vi "BESS reconnect.vi"() -> (1 "failure_flag 2":bool)   [LabVIEW 2016]
uses:
  Communication/Global communication.vi
  Communication/Global communication output.vi
panel:
  in  "ready?":bool
  in  "i>=20?":bool
  in  "=1?":bool
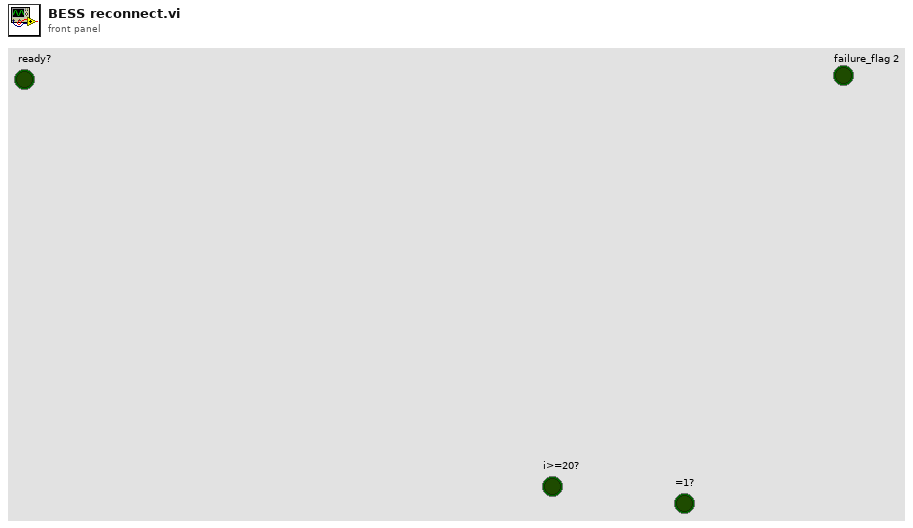
[diagram p1: front panel]
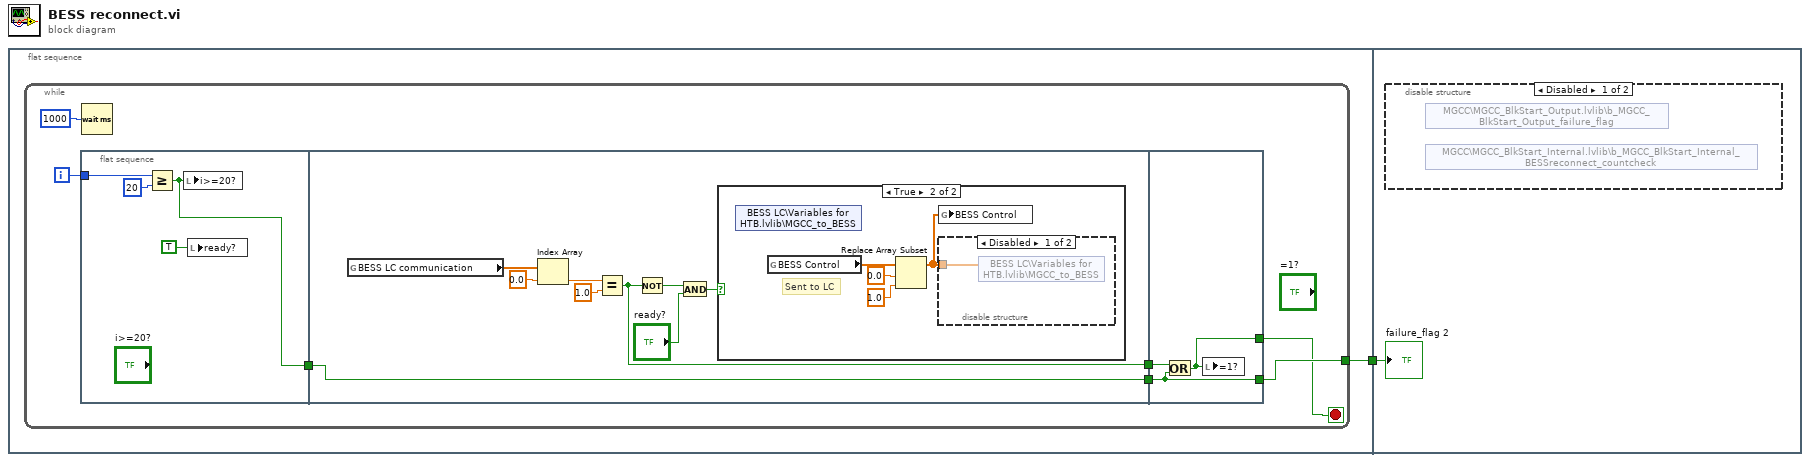
[diagram p0: block diagram]
diagram:
  n1 = flat-sequence {
    tunnel: [w2] -> w1
    tunnel: w1 -> [w31]
    frame #0 {
      n2 = while {
        tunnel: [w4] -> w2
        i -> [w8]
        stop <- w3 stop-if-true
        n3 = flat-sequence {
          tunnel: w8 -> [w13]
          tunnel: [w10] -> w7
          tunnel: w7 -> [w21]
          tunnel: [w21] -> w6
          tunnel: [w17] -> w5
          tunnel: w6 -> [w29]
          tunnel: w5 -> [w30]
          tunnel: [w29] -> w4
          tunnel: [w28] -> w3
          frame #0 {
            n4 = Greater Or Equal?(x=w13, y=20) -> (x >= y?=w10:bool)
            n5 = local write "i>=20?"(w10) -> ()
            n6 = local write "ready?"(TRUE) -> ()
          }
          frame #1 {
            n7 = global read "Global communication.vi" "BESS LC communication"() -> (w14:dbl[])
            n8 = Index Array(array=w14, index=0.0) -> (element=w15:dbl)
            n9 = Equal?(x=w15, y=1.0) -> (x = y?=w17:bool)
            n10 = Not(x=w17) -> (.not. x?=w19:bool)
            n11 = And(x=w19, y="ready?") -> (x .and. y?=w20:bool)
            n12 = case shown="True" w20 {
              frame False {
              }
              frame True {
                # "Sent to LC"
                n13 = shared-variable "BESS LC\\Variables for HTB.lvlib\\MGCC_to_BESS"() -> ()  [unwired: 1 in, 2 out]
                n14 = global read "Global communication output.vi" "BESS Control"() -> (w24:dbl[])
                n15 = Replace Array Subset(array=w24, new element=1.0, index=0.0) -> (w23:dbl[])
                n16 = global write "Global communication output.vi" "BESS Control"(w23) -> ()
                n17 = disable-structure shown="Disabled" {
                  disable-tunnel: w23 -> [w27 _]
                  frame Disabled {
                    n18 = shared-variable "BESS LC\\Variables for HTB.lvlib\\MGCC_to_BESS"(w27) -> ()  [unwired: 1 in, 1 out]
                  }
                  frame Enabled {
                  }
                }
              }
            }
          }
          frame #2 {
            n19 = Or(x=w30, y=w29) -> (x .or. y?=w28:bool)
            n20 = local write "=1?"(w28) -> ()
          }
        }
        n21 = Wait (ms)(milliseconds to wait=1000) -> ()  [unwired: 1 out]
      }
    }
    frame #1 {
      n22 = disable-structure shown="Disabled" {
        frame Disabled {
          n23 = shared-variable "MGCC\\MGCC_BlkStart_Output.lvlib\\b_MGCC_BlkStart_Output_failure_flag"() -> ()  [unwired: 2 in, 1 out]
          n24 = shared-variable "MGCC\\MGCC_BlkStart_Internal.lvlib\\b_MGCC_BlkStart_Internal_BESSreconnect_countcheck"() -> ()  [unwired: 1 in, 2 out]
        }
        frame Enabled {
        }
      }
      "failure_flag 2" <- w31
    }
  }
